vi "Qrcode YGB Complete.vi"() -> ()   [LabVIEW 2019]
uses:
  <vilib>/userDefined/High Color/IMAQdx.ctl
  <vilib>/vision/driver/NI_Vision_Acquisition_Software.lvlib
  <vilib>/vision/NI_Vision_Development_Module.lvlib
panel:
  out "sorted array":string[](array[string])
  out "Blue":bool
  out "Green":bool
  out "Yellow":bool
  out "Array 2":string[](array[string])
  out "element 3":string
  out "element 2":string
  out "element":string
  out "Codes":string[](array[string])
  out "Found?":bool
  out "Image":T1(plugin-control)
  out "Data":string
  in  "Session In":T2
  out "Numeric":dbl
  out "Enum":enum16{"scan", "execute"}(ring)
  in  "Array":T3(array[cluster])
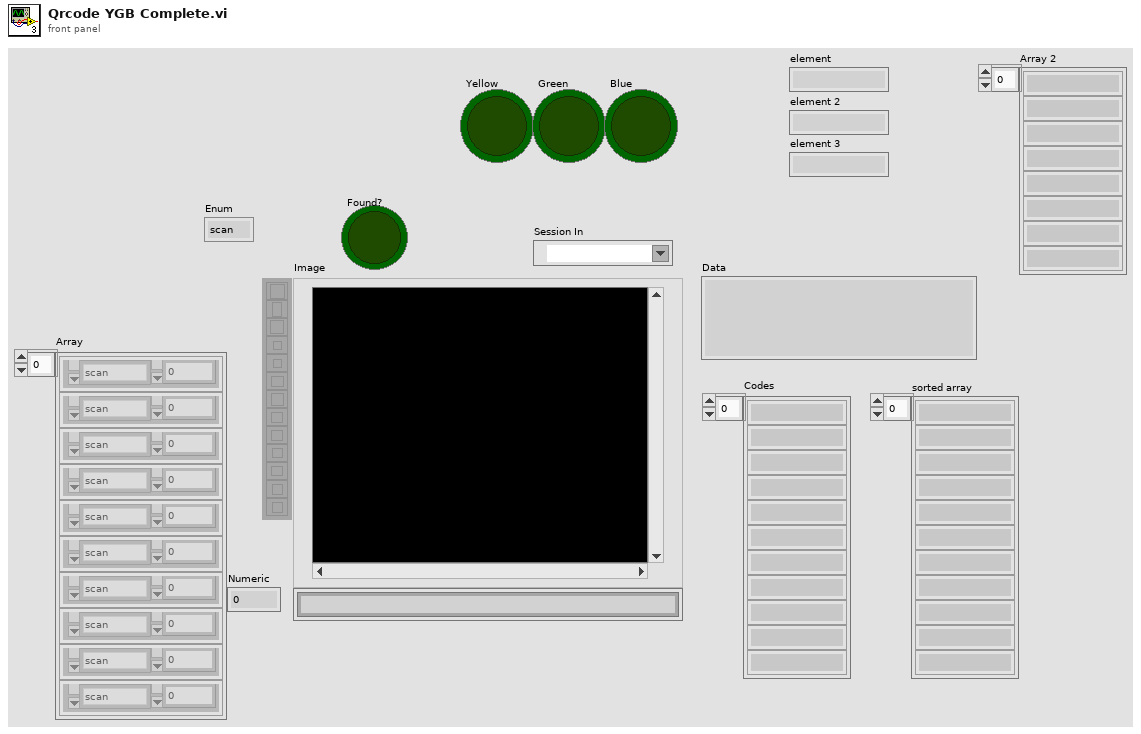
[diagram p1: front panel]
types:
  T1 = typedef "IMAQ Image.ctl" = refnum<image>
  T2 = typedef "IMAQdx.ctl" = refnum<k21>
  T3 = cluster{"Enum":enum16{"scan", "execute"}, "Numeric":dbl}[]
  T4 = typedef "Image Type" = u32
  T5 = typedef "QR Code Report.ctl" = cluster{"Found?":bool, "Data":string, "Bounding Box":cluster{"x":sgl, "y":sgl}[], "Errors Corrected":u32, "Dimensions (Rows/Cols)":u32, "Version":u32, "QR Model":T6, "Stream Mode":T7, "Barcode Polarity":T8, "Mirrored?":bool, "Append Stream Position":u32, "Size of Append Stream":u32, "First EAN-128 ID":i32, "First Alternate Language ID":i32, "Append Stream ID":u32, "Minimum Edge Strength":u32, "Demodulation Mode":T9, "Cell Sample Size":T10, "Cell Filter Mode":T11}
  T6 = typedef "QR Code Model Type.ctl" = i32
  T7 = typedef "QR Code Stream Mode Type.ctl" = i32
  T8 = typedef "Data Matrix Polarity.ctl" = i32
  T9 = typedef "Demodulation Mode.ctl" = i32
  T10 = typedef "Cell Sample Size.ctl" = i32
  T11 = typedef "Cell Filter Mode.ctl" = i32
  T12 = cluster{"Enum":enum16{"scan", "execute"}, "Numeric":dbl}
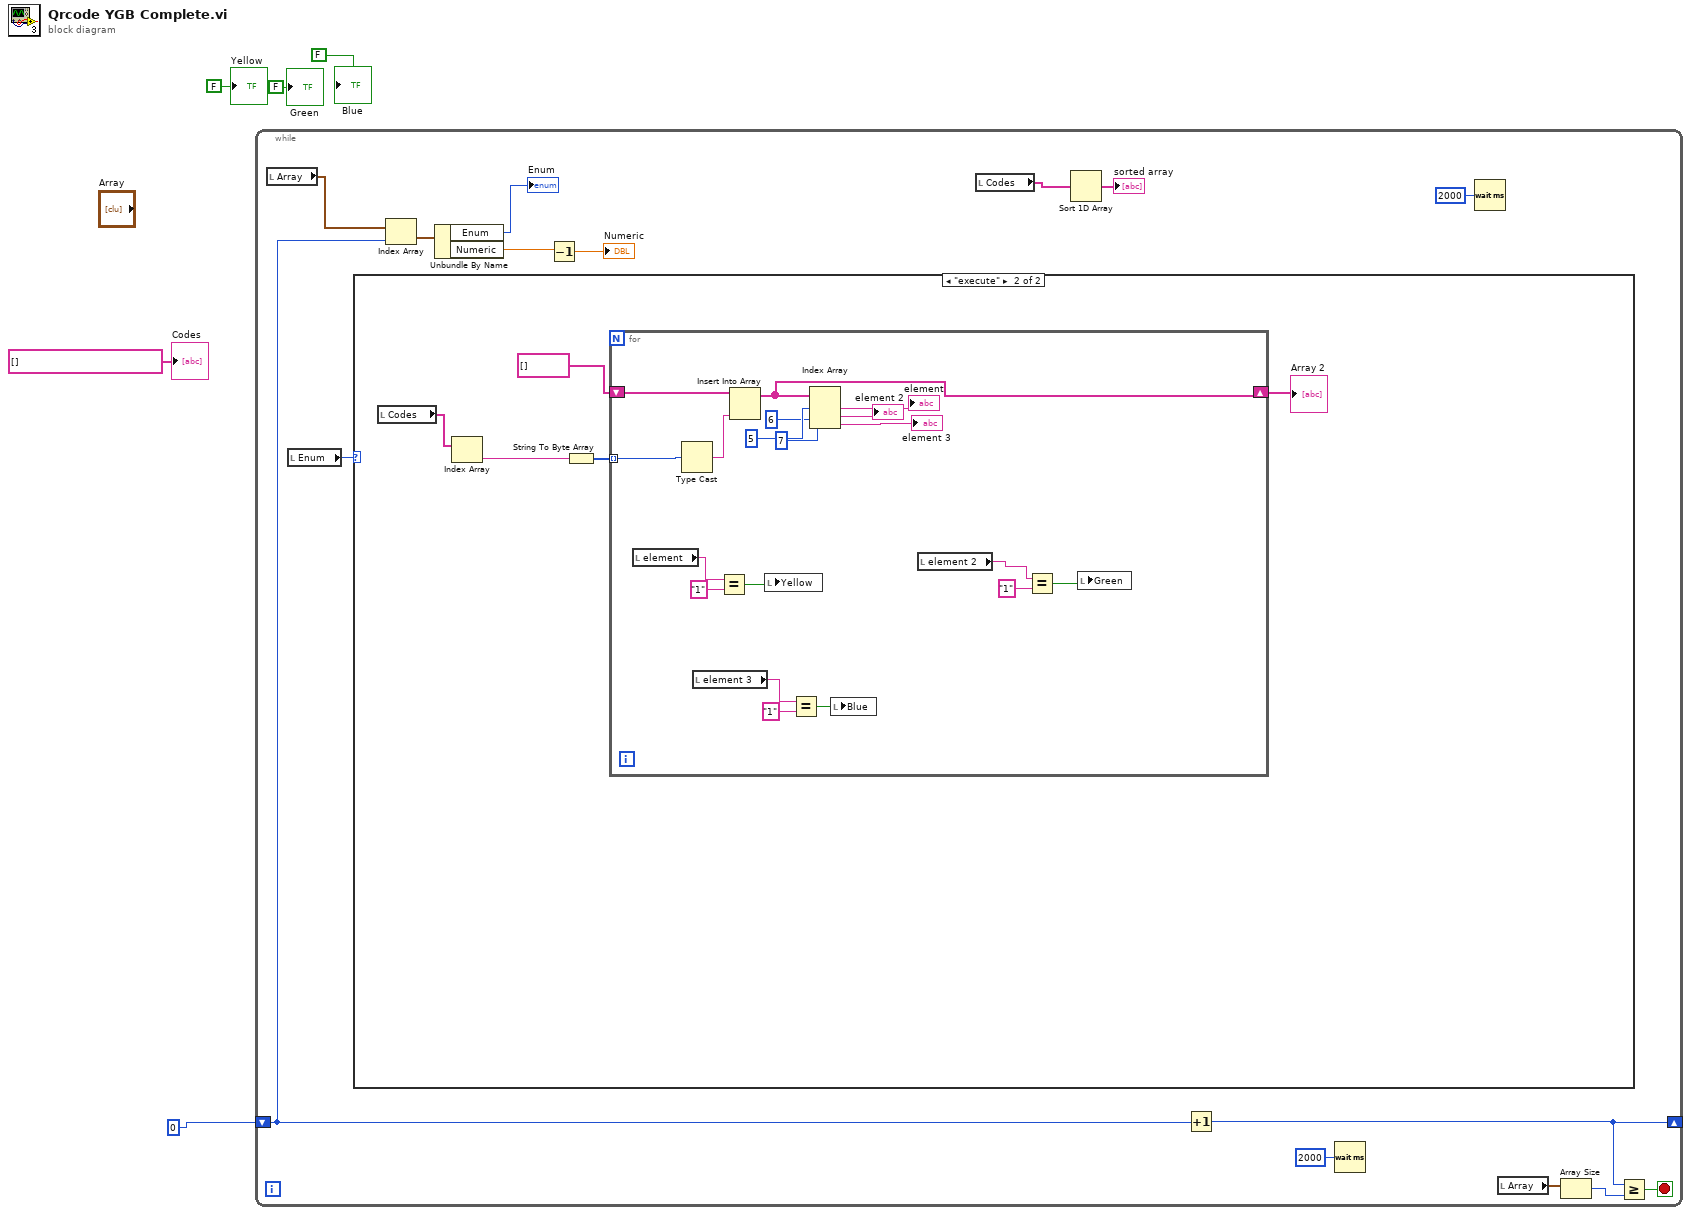
[diagram p0: block diagram]
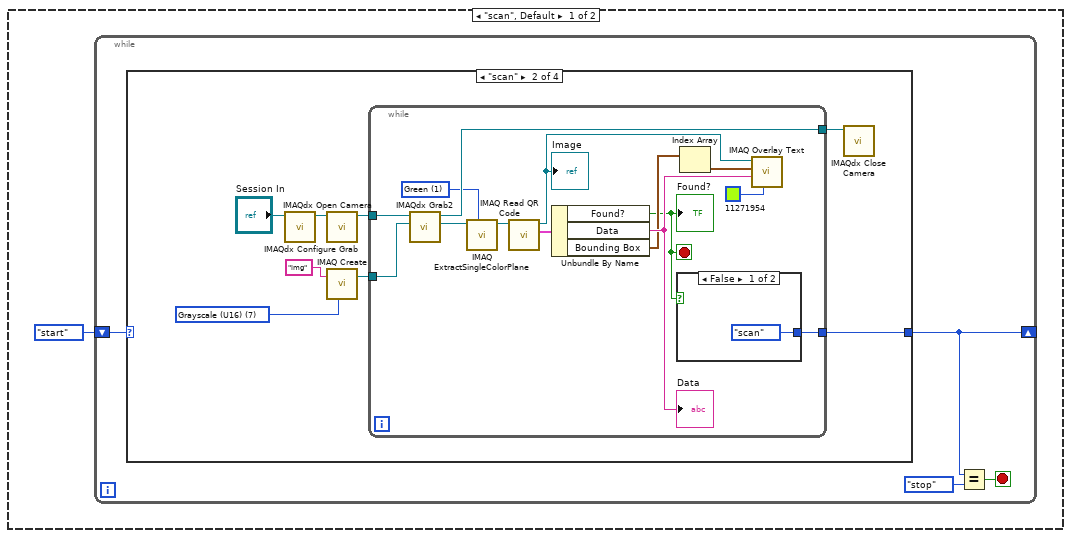
[diagram p2: hidden frame]
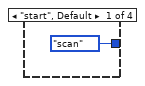
[diagram p3: hidden frame]
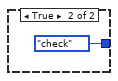
[diagram p4: hidden frame]
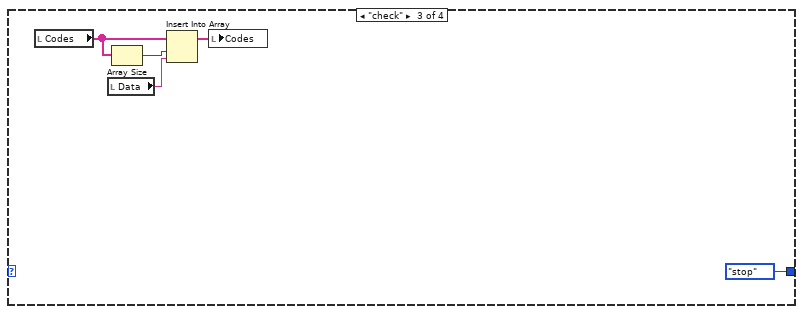
[diagram p5: hidden frame]
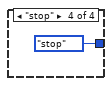
[diagram p6: hidden frame]
diagram:
  n1 = while {
    shift-right: [w17] -> _
    shift-left: 0 -> [w19]
    stop <- w18 stop-if-true
    n2 = local read "Array"() -> (w16:T3)
    n3 = local read "Enum"() -> (w11:enum16{"scan", "execute"})
    n4 = case shown="\"execute\"" w11 {
      frame "scan", Default {
        n5 = while {
          shift-right: [w22] -> _
          shift-left: enum16{"start", "scan", "check", "stop"}."start" -> [w25]
          stop <- w23 stop-if-true
          n6 = case shown="\"scan\"" w25 {
            tunnel: [enum16{"start", "scan", "check", "stop"}."scan" w27 enum16{"start", "scan", "check", "stop"}."stop" enum16{"start", "scan", "check", "stop"}."stop"] -> w22
            frame "start", Default {
            }
            frame "scan" {
              w29 = T4 7 items=["Grayscale (U8)", "Grayscale (I16)", "Grayscale (SGL)", "Complex (CSG)", "RGB (U32)", "HSL (U32)", "RGB (U64)", "Grayscale (U16)"] ("Image Type")
              n7 = call <vilib>:"IMAQdx Open Camera.vi"("Session In"="Session In") -> ("Session Out"=w33:T2)  [unwired: 9 in, 1 out]
              n8 = call <vilib>:"IMAQdx Configure Grab.vi"("Session In"=w33) -> ("Session Out"=w31:T2)  [unwired: 9 in, 1 out]
              n9 = call "IMAQ Create"("Image Name"="img", "Image Type"=w29) -> ("New Image"=w28:T1)  [unwired: 3 in, 1 out]
              n10 = while {
                tunnel: [w48] -> w32
                tunnel: w31 -> [w47]
                tunnel: w28 -> [w46]
                tunnel: [w35] -> w27
                stop <- w36 stop-if-true
                w43 = 1 items=["Red", "Green", "Blue", "Hue", "Saturation", "Luminance", "Value", "Intensity"] ("Color Plane")
                n11 = call <vilib>:"IMAQdx Grab2.vi"("Image In"=w46, "Session In"=w47) -> ("Image Out"=w45:T1, "Session Out"=w48:T2)  [unwired: 6 in, 2 out]
                n12 = call "IMAQ ExtractSingleColorPlane"("Color Plane"=w43, "Image Src"=w45) -> ("Image Dst Out"=w44:T1)  [unwired: 8 in, 1 out]
                n13 = call "IMAQ Read QR Code"("Image"=w44) -> ("QR Code Report"=w42:T5, "Image (duplicate)"=w37:T1)  [unwired: 7 in, 2 out]
                "Image" <- w37
                n14 = Unbundle By Name(w42) -> ("Found?"=w36:bool, "Data"=w40:string, "Bounding Box"=w38:cluster{"x":sgl, "y":sgl}[])
                "Found?" <- w36
                "Data" <- w40
                n15 = case shown="False" w36 {
                  tunnel: [enum16{"start", "scan", "check", "stop"}."scan" enum16{"start", "scan", "check", "stop"}."check"] -> w35
                  frame False {
                  }
                  frame True {
                  }
                }
                n16 = Index Array(array=w38) -> (element=w41:cluster{"x":sgl, "y":sgl})  [unwired: 1 in]
                n17 = call "IMAQ Overlay Text"("Text Color (black)"=u32 11271954, "String"=w40, "Origin"=w41, "Image"=w37) -> ()  [unwired: 6 in, 2 out]
              }
              n18 = call <vilib>:"IMAQdx Close Camera.vi"("Session In"=w32) -> ()  [unwired: 10 in, 1 out]
            }
            frame "check" {
              n19 = local read "Codes"() -> (w55:string[])
              n20 = local read "Data"() -> (w53:string)
              n21 = Array Size(array=w55) -> (size(s)=w54:i32)
              n22 = Insert Into Array(array=w55, index=w54, new element=w53) -> (w52:string[])
              n23 = local write "Codes"(w52) -> ()
            }
            frame "stop" {
            }
          }
          n24 = Equal?(x=w22, y=enum16{"start", "scan", "check", "stop"}."stop") -> (x = y?=w23:bool)
        }
      }
      frame "execute" {
        n25 = local read "Codes"() -> (w61:string[])
        n26 = Index Array(array=w61) -> (element=w60:string)  [unwired: 1 in]
        n27 = String To Byte Array(string=w60) -> (unsigned byte array=w59:u8[])
        n28 = for {
          tunnel: w59 -> [w80] mode=indexing
          shift-right: [w71] -> w57
          shift-left: string[] [] -> [w79]
          n29 = local read "element"() -> (w70:string)
          n30 = Type Cast(x=w80) -> (*(type *) &x=w78:string)  [unwired: 1 in]
          n31 = local read "element 3"() -> (w66:string)
          n32 = Equal?(x=w70, y="1") -> (x = y?=w64:bool)
          n33 = Insert Into Array(array=w79, new element=w78) -> (w71:string[])  [unwired: 1 in]
          n34 = local write "Yellow"(w64) -> ()
          n35 = Equal?(x=w66, y="1") -> (x = y?=w63:bool)
          n36 = Index Array(array=w71, index #1=5 ("index"), index #2=6 ("index"), index #3=7 ("index")) -> (element #1=→"element":string, element #2=→"element 2":string, element #3=→"element 3":string)
          n37 = local write "Blue"(w63) -> ()
          n38 = local read "element 2"() -> (w68:string)
          n39 = Equal?(x=w68, y="1") -> (x = y?=w62:bool)
          n40 = local write "Green"(w62) -> ()
        }
        "Array 2" <- w57
      }
    }
    n41 = Index Array(array=w16, index=w19) -> (element=w13:T12)
    n42 = Unbundle By Name(w13) -> ("Enum"=→"Enum":enum16{"scan", "execute"}, "Numeric"=w9:dbl)
    n43 = Decrement(x=w9) -> (x-1=→"Numeric":dbl)
    n44 = local read "Codes"() -> (w7:string[])
    n45 = Sort 1D Array(array=w7) -> (sorted array=→"sorted array":string[])
    n46 = Increment(x=w19) -> (x+1=w17:i32)
    n47 = Wait (ms)(milliseconds to wait=u32 2000) -> ()  [unwired: 1 out]
    n48 = Wait (ms)(milliseconds to wait=u32 2000) -> ()  [unwired: 1 out]
    n49 = local read "Array"() -> (w14:T3)
    n50 = Array Size(array=w14) -> (size(s)=w15:i32)
    n51 = Greater Or Equal?(x=w17, y=w15) -> (x >= y?=w18:bool)
  }
  "Codes" <- string[] [] ("Array 2")
  "Yellow" <- FALSE ("Yellow")
  "Green" <- FALSE ("Green")
  "Blue" <- FALSE ("Blue")
